vi "Vision Processing.vi"(4 "error in (no error)":errorcluster, 7 "Image Size":T1=enum."160x120") -> ()   [LabVIEW 2016]
doc: "This VI runs in parallel to other tasks. It gets images from the camera, processes them for color or shape and use that information to affect robot behavior."
uses:
  <vilib>/Rock Robotics/WPI/Camera/WPI_CameraImageSize.ctl
  <vilib>/Rock Robotics/WPI/Camera/WPI_CameraWhite Balance Values.ctl
  <vilib>/Rock Robotics/WPI/Camera/WPI_CameraFrameRate.ctl
  <vilib>/Rock Robotics/WPI/Camera/WPI_CameraExposure Values.ctl
  Robot Global Data.vi
  AutoaimVar.vi
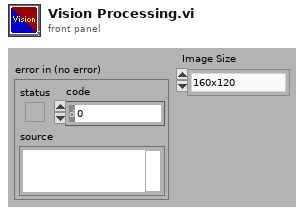
[diagram p1: front panel]
types:
  T1 = typedef "WPI_CameraImageSize.ctl" = enum16{"640x480", "320x240", "160x120", "Custom"}
  T2 = typedef "WPI_CameraExposure Values.ctl" = enum16{"Auto", "Flicker-free 50 Hz", "Flicker-free 60 Hz", "Hold current", "Custom"}
  T3 = typedef "Image Type" = u32
  T4 = typedef "WPI_CameraFrameRate.ctl" = u32
  T5 = typedef "WPI_CameraWhite Balance Values.ctl" = enum16{"Auto", "Fixed indoor", "Fixed outdoor 1", "Fixed outdoor 2", "Fixed fluorescent 1", "Fixed fluorescent 2", "Hold current", "Custom"}
  T6 = typedef "WPI_CameraDevRef.ctl" = cluster{"Camera Address":string, "CameraStatus":errorcluster}
  T7 = typedef "IMAQ Image.ctl" = refnum<image>
  T8 = typedef "WPI_GyroDevRef.ctl" = cluster{"DevStatus":errorcluster, "Analog Channel":T9, "Offset":dbl, "Gain (VoltsPerDegree/Second)":dbl, "Gyro Type":enum16{"Analog", "XRS450"}, "Handle":i32, "SPI Bus":T10, "Device Found":bool, "Sample Rate":dbl, "Calibrate On Open":bool}
  T9 = typedef "FPGA_AIChannel.ctl" = enum8{"AI 0", "AI 1", "AI 2", "AI 3", "AI MXP 0", "AI MXP 1", "AI MXP 2", "AI MXP 3", "Invalid"}
  T10 = typedef "spi_bus.ctl" = enum16{"SPI On-Board, CS0", "SPI On-Board, CS1", "SPI On-Board, CS2", "SPI On-Board, CS3", "SPI MXP", "Invalid"}
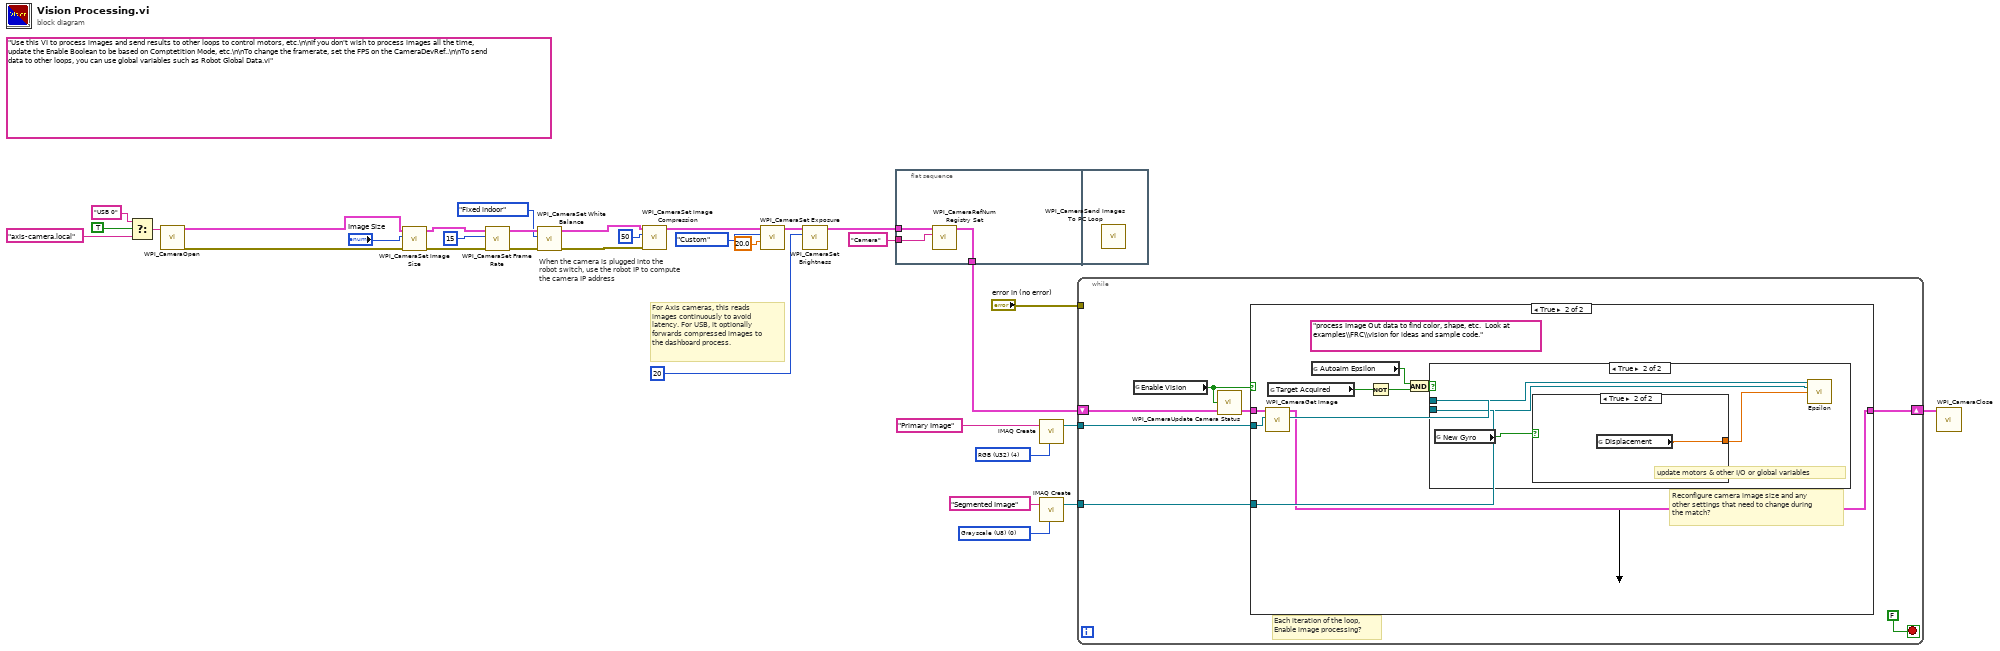
[diagram p0: block diagram]
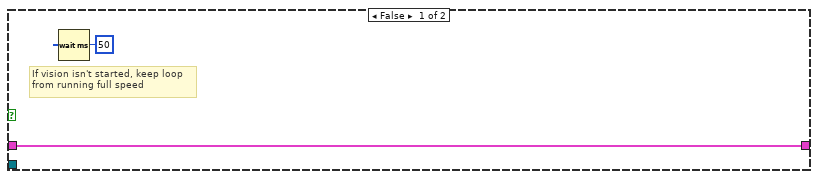
[diagram p2: hidden frame]
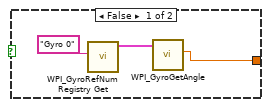
[diagram p4: hidden frame]
diagram:
  w11 = T3 0 items=["Grayscale (U8)", "Grayscale (I16)", "Grayscale (SGL)", "Complex (CSG)", "RGB (U32)", "HSL (U32)", "RGB (U64)"] ("Image Type")
  (unwired) "Use this VI to process images and send results to other loops to control motors, etc.\n\nIf you don't wish to process images all the time, update the Enable Boolean to be based on Comptetition Mode, etc.\n\nTo change the framerate, set the FPS on the CameraDevRef..\n\nTo send data to other loops, you can use global variables such as Robot Global Data.vi"
  w32 = T3 4 items=["Grayscale (U8)", "Grayscale (I16)", "Grayscale (SGL)", "Complex (CSG)", "RGB (U32)", "HSL (U32)", "RGB (U64)"] ("Image Type")
  # "When the camera is plugged into the\nrobot switch, use the robot IP to compute\nthe camera IP address"
  # "For Axis cameras, this reads\nimages continuously to avoid\nlatency. For USB, it optionally\nforwards compressed images to\nthe dashboard process."
  n1 = Select(t="USB 0" ("format string"), s=TRUE ("dot notation? (F)"), f="axis-camera.local" ("format string")) -> (s? t:f=w15:string)
  n2 = call <vilib>:"WPI_CameraOpen.vi"("Camera Address"=w15) -> ("error out"=w25:errorcluster, "CameraDevRef"=w26:T6)  [unwired: 1 in, 8 out]
  n3 = call <vilib>:"WPI_CameraSet Image Size.vi"("error in (no error)"=w25, "Image Size"="Image Size", "CameraDevRef"=w26) -> ("error out"=w24:errorcluster, "CameraDevRef Out"=w27:T6)  [unwired: 1 in, 6 out]
  n4 = call <vilib>:"WPI_CameraSet Frame Rate.vi"("error in (no error)"=w24, "Frame Rate (fps)"=T4 15, "CameraDevRef"=w27) -> ("error out"=w23:errorcluster, "CameraDevRef Out"=w28:T6)  [unwired: 7 out]
  n5 = call <vilib>:"WPI_CameraSet White Balance.vi"("error in (no error)"=w23, "White Balance"=WPI_CameraWhite_Balance_Values."Fixed indoor", "CameraDevRef"=w28) -> ("error out"=w9:errorcluster, "CameraDevRef Out"=w10:T6)  [unwired: 1 in, 6 out]
  n6 = call <vilib>:"WPI_CameraSet Image Compression.vi"("error in (no error)"=w9, "Compression"=50, "CameraDevRef"=w10) -> ("CameraDevRef Out"=w6:T6)  [unwired: 8 out]
  n7 = call <vilib>:"WPI_CameraSet Exposure.vi"("Exposure (%)"=20.0, "Exposure"=WPI_CameraExposure_Values."Custom", "CameraDevRef"=w6) -> ("CameraDevRef Out"=w5:T6)  [unwired: 1 in, 7 out]
  n8 = call <vilib>:"WPI_CameraSet Brightness.vi"("Brightness"=20, "CameraDevRef"=w5) -> ("CameraDevRef Out"=w3:T6)  [unwired: 1 in, 8 out]
  n9 = flat-sequence {
    tunnel: w3 -> [w35]
    tunnel: "Camera" ("refnum name") -> [w34]
    tunnel: [w33] -> w1
    frame #0 {
      n10 = call <vilib>:"WPI_CameraRefNum Registry Set.vi"("refnum name"=w34, "CameraDevRef"=w35) -> ("CameraDevRef"=w33:T6)  [unwired: 2 in, 7 out]
    }
    frame #1 {
      n11 = call <vilib>:"WPI_CameraSend Images To PC Loop.vi"() -> ()  [unwired: 12 in]
    }
  }
  n12 = call "IMAQ Create"("Image Name"="Primary Image", "Image Type"=w32) -> ("New Image"=w30:T7)  [unwired: 2 in, 2 out]
  n13 = call "IMAQ Create"("Image Name"="Segmented Image", "Image Type"=w11) -> ("New Image"=w12:T7)  [unwired: 2 in, 2 out]
  n14 = while {
    shift-right: [w41] -> w19
    shift-left: w1 -> [w39]
    tunnel: w30 -> [w40]
    tunnel: "error in (no error)" -> [_]
    tunnel: w12 -> [w36]
    stop <- FALSE stop-if-true
    # "Each iteration of the loop,\nEnable image processing?"
    n15 = global read "Robot Global Data.vi" "Enable Vision"() -> (w37:bool)
    n16 = call <vilib>:"WPI_CameraUpdate Camera Status.vi"("CameraDevRef In"=w39, "Enable Vision"=w37) -> ("CameraDevRef Out"=w38:T6)  [unwired: 3 in]
    n17 = case shown="True" w37 {
      tunnel: w40 -> [_ w53]
      tunnel: [w44 w45] -> w41
      tunnel: w38 -> [w44 w52]
      tunnel: w36 -> [_ w50]
      frame False {
        # "If vision isn't started, keep loop\nfrom running full speed"
        n18 = Wait (ms)(milliseconds to wait=u32 50) -> ()  [unwired: 1 out]
      }
      frame True {
        (unwired) "process Image Out data to find color, shape, etc.  Look at examples\\FRC\\vision for ideas and sample code."
        # "Reconfigure camera image size and any\nother settings that need to change during\nthe match?"
        n19 = call <vilib>:"WPI_CameraGet Image.vi"("Image"=w53, "CameraDevRef"=w52) -> ("Image Out"=w51:T7, "CameraDevRef Out"=w45:T6)  [unwired: 1 in, 7 out]
        n20 = global read "AutoaimVar.vi" "Target Acquired"() -> (w49:bool)
        n21 = global read "AutoaimVar.vi" "Autoaim Epsilon"() -> (w47:bool)
        n22 = Not(x=w49) -> (.not. x?=w48:bool)
        n23 = And(x=w47, y=w48) -> (x .and. y?=w46:bool)
        n24 = case shown="True" w46 {
          tunnel: w51 -> [_ w57]
          tunnel: w50 -> [_ w56]
          frame False {
          }
          frame True {
            # "update motors & other I/O or global variables"
            n25 = global read "Robot Global Data.vi" "New Gyro"() -> (w55:bool)
            n26 = case shown="True" w55 {
              tunnel: [w58 w61] -> w54
              frame False {
                n27 = call <vilib>:"WPI_GyroRefNum Registry Get.vi"("refnum name"="Gyro 0") -> ("GyroDevRef"=w59:T8)  [unwired: 9 in, 1 out]
                n28 = call <vilib>:"WPI_GyroGetAngle.vi"("GyroDevRef"=w59) -> ("Angle"=w58:dbl)  [unwired: 6 in, 4 out]
              }
              frame True {
                n29 = global read "Robot Global Data.vi" "Displacement"() -> (w61:dbl)
              }
            }
            n30 = call "Epsilon.vi"("Image"=w57, "SegImg"=w56, "Gyro Position"=w54) -> ()  [unwired: 13 in]
          }
        }
      }
    }
  }
  n31 = call <vilib>:"WPI_CameraClose.vi"("CameraDevRef"=w19) -> ()  [unwired: 1 in, 10 out]
